vi "Write Setting File Data.vi"(0 "VISA resource name":refnum<visa-resource-name>, 7 "Setting File Name (\"\")":path, 11 "error in (no error)":errorcluster) -> (4 "VISA resource name out":refnum<visa-resource-name>, 15 "error out":errorcluster)   [LabVIEW 2020, in "Yokogawa GX Series.lvlib"]
doc: "Sends the setting data in the file for configuration."
uses:
  <instrlib>/Yokogawa GX Series/Yokogawa GX Series.lvlib
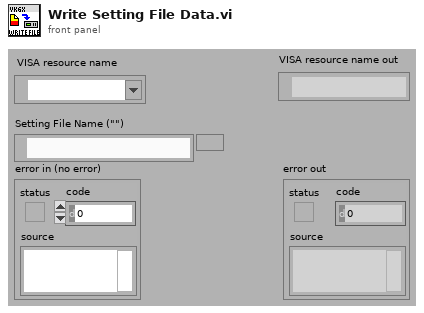
[diagram p1: front panel]
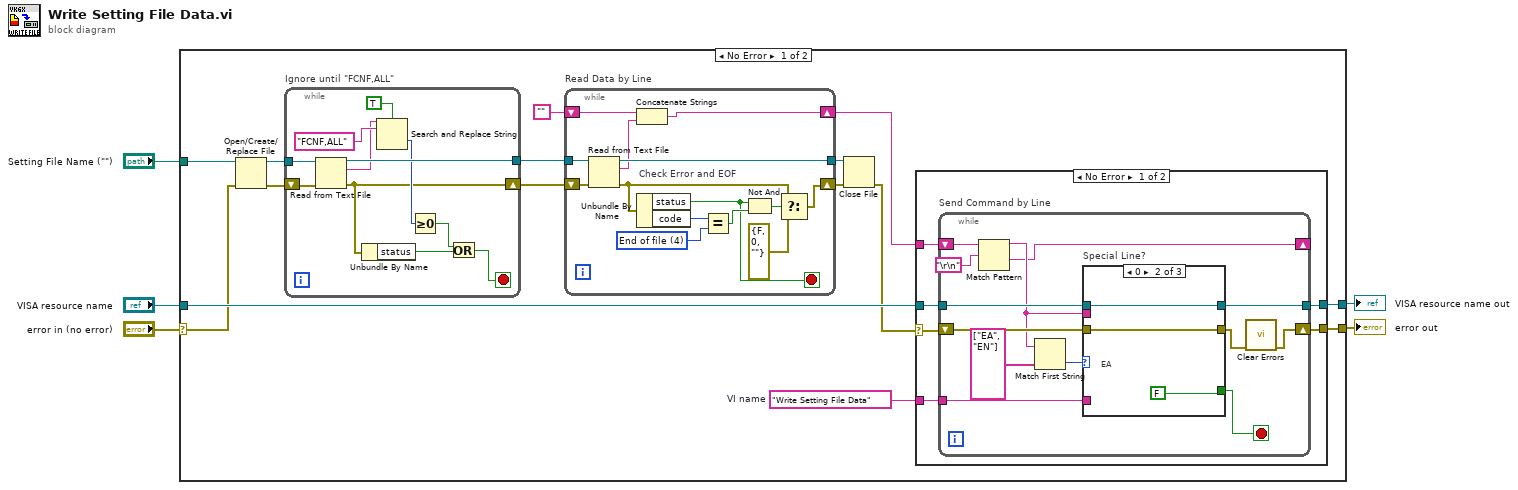
[diagram p0: block diagram]
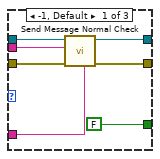
[diagram p2: hidden frame]
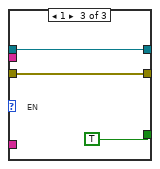
[diagram p3: hidden frame]
diagram:
  n1 = case shown="No Error" "error in (no error)" {
    selector: "error in (no error)" -> [w7 w80]
    tunnel: "Setting File Name (\"\")" -> [w20 _]
    tunnel: "VISA resource name" -> [w10 w81]
    tunnel: [w9 w81] -> w3
    tunnel: [w8 w80] -> w2
    frame No Error {
      w11 = "Write Setting File Data"  # VI name
      n2 = Open/Create/Replace File(file path (use dialog)=w20, error in=w7) -> (refnum out=w19:refnum<file>, error out=w18:errorcluster)  [unwired: 4 in, 1 out]
      n3 = while "Ignore until \"FCNF,ALL\"" {
        tunnel: w19 -> [w65]
        tunnel: [w63] -> w17
        shift-right: [w58] -> w16
        shift-left: w18 -> [w64]
        stop <- w56 stop-if-true
        n4 = Read from Text File(file (use dialog)=w65, error in=w64) -> (refnum out=w63:refnum<file>, text=w59:string, error out=w58:errorcluster)  [unwired: 2 in, 1 out]
        n5 = Unbundle By Name(w58) -> ("status"=w55:bool)
        n6 = Search and Replace String(case sensitive?=TRUE, input string=w59, search string="FCNF,ALL") -> (offset past replacement=w61:i32)  [unwired: 5 in, 3 out]
        n7 = Greater Or Equal To 0?(x=w61) -> (x >= 0?=w57:bool)
        n8 = Or(x=w57, y=w55) -> (x .or. y?=w56:bool)
      }
      n9 = while "Read Data by Line" {
        shift-left: "" -> [w76]
        shift-right: [w75] -> w12
        shift-left: w16 -> [w78]
        shift-right: [w69] -> w15
        tunnel: w17 -> [w79]
        tunnel: [w77] -> w14
        stop <- w68 stop-if-true
        w66 = 4 items=["No error", "Argument error", "Memory is full", "Out of zone", "End of file", "File already open", "Generic file I/O error", "File not found", "File permission error", "Disk is full", "Duplicate path", "Too many files open", "System feature not enabled", "Resource file not found", "Cannot add resource", "Resource not found", "Image not found", "Image memory error", "Pen does not exist", "Config type invalid", "Config token not found", "Config parse error", "Config memory error", "Bad external code format", "Bad external code offset", "External code not present", "Null window", "Destroy window error", "Null menu", "Print aborted", "Bad print record", "Print driver error", "Windows error during printing", "Memory error during printing", "Print dialog error", "Generic print error", "Invalid device refnum", "Device not found", "Device parameter error", "Device unit error", "Cannot open device", "Device call aborted", "Generic error", "Cancelled by user", "Object ID too low", "Object ID too high", "Object not in heap", "Unknown heap", "Unknown object (invalid DefProc)", "Unknown object (DefProc not in table)", "Message out of range", "Invalid (null) method", "Unknown message", "Manager call not supported", "Bad address", "Network operation in progress", "Network operation timed out", "Connection is busy", "Network attribute not supported", "Network error", "Address in use", "System out of memory", "Connection aborted", "Connection refused", "Not connected", "Already connected", "Connection closed", "Initialization error (interapplication manager)", "Bad occurrence", "Wait on unbound occurrence handler", "Occurrence queue overflow", "Datalog type conflict", "Unused", "Unrecognized type (interapplication manager)", "Memory corrupt", "Failed to make temporary DLL", "Old CIN version", "Drag socket not found", "Failed to load drop-object", "Failed to register OLE object", "Failed to release OLE object", "Format specifier type mismatch", "Unknown format specifier", "Too few format specifiers", "Too many format specifiers", "Scan failed", "Unknown error code"]
        # "Check Error and EOF"
        n10 = Read from Text File(file (use dialog)=w79, error in=w78) -> (refnum out=w77:refnum<file>, text=w74:string, error out=w70:errorcluster)  [unwired: 3 out]
        n11 = Concatenate Strings(w76, w74) -> (w75:string)
        n12 = Unbundle By Name(w70) -> ("status"=w68:bool, "code"=w73:i32)
        n13 = Equal?(x=w73, y=w66) -> (x = y?=w72:bool)
        n14 = Not And(1:w72, 2:w68) -> (0:w71:bool)
        n15 = Select(t=w70, s=w71, f=errorcluster {FALSE, 0, ""} ("出力クラスタ")) -> (s? t:f=w69:errorcluster)
      }
      n16 = Close File(refnum=w14, error in=w15) -> (error out=w6:errorcluster)  [unwired: 1 out]
      n17 = case shown="No Error" w6 {
        selector: w6 -> [w21 w53]
        tunnel: w12 -> [w26 _]
        tunnel: w11 -> [w25 _]
        tunnel: w10 -> [w24 w54]
        tunnel: [w23 w54] -> w9
        tunnel: [w22 w53] -> w8
        frame No Error {
          n18 = while "Send Command by Line" {
            shift-left: w21 -> [w38]
            shift-right: [w27] -> w22
            shift-left: w26 -> [w39]
            shift-right: [w33] -> _
            tunnel: w25 -> [w34]
            tunnel: w24 -> [w37]
            tunnel: [w36] -> w23
            stop <- w29 stop-if-true
            n19 = Match Pattern(string=w39, regular expression="\r\n") -> (before substring=w35:string, after substring=w33:string)  [unwired: 3 out]
            n20 = Match First String(2:string[] ["EA", "EN"], 3:w35) -> (0:w32:i32)  [unwired: 1 out]
            n21 = case "Special Line?" shown="0" w32 {
              tunnel: w37 -> [w46 w49 w52]
              tunnel: w38 -> [w44 w48 w51]
              tunnel: [w42 w48 w51] -> w28
              tunnel: [w41 w49 w52] -> w36
              tunnel: w35 -> [w45 _ _]
              tunnel: w34 -> [w43 _ _]
              tunnel: [FALSE FALSE TRUE] -> w29
              frame -1, Default {
                n22 = call <instrlib>:"Send Message Normal Check.vi"("Source (\"\")"=w43, "error in (no error)"=w44, "Send Message (\"\")"=w45, "VISA resource name"=w46) -> ("error out"=w42:errorcluster, "VISA resource name out"=w41:refnum<visa-resource-name>)  [unwired: 1 in, 5 out]
              }
              frame 0 {
                # "EA"
              }
              frame 1 {
                # "EN"
              }
            }
            n23 = call <vilib>:"Clear Errors.vi"("error in (no error)"=w28) -> ("error out"=w27:errorcluster)  [unwired: 5 in, 1 out]
          }
        }
        frame Error {
        }
      }
    }
    frame Error {
    }
  }
  "error out" <- w2
  "VISA resource name out" <- w3
